vi "Do.vi"(8 "error in (no error)":errorcluster, 10 "Actor in":refnum<class "Actor.lvclass">, 11 "Return Run VI State Msg":refnum<class "Return Run VI State Msg.lvclass">) -> (0 "error out":errorcluster, 2 "Actor out":refnum<class "Actor.lvclass">)   [LabVIEW 2013, in "tWorkerTCPConnection.lvlib" / "Return Run VI State Msg.lvclass"]
doc: "(<B>Filename</B>: Actor Framework.lvlib:Message.lvclass:Do.vi)\n\nDefines what a message does when it is received by an actor. Generally, a message instructs an actor to invoke one of its methods.\n\nBy default, this method does nothing. A child class must override it to define behavior. Create a child class by using the Actor Framework Message Maker dialog box."
uses:
  Return Run VI State Msg.lvclass
  <vilib>/ActorFramework/Actor/Actor.lvclass
  tWorkerTCPConnection/tWorkerTCPConnection.lvclass
  Return Run VI State Msg.lvclass/Return Run VI State Msg.ctl
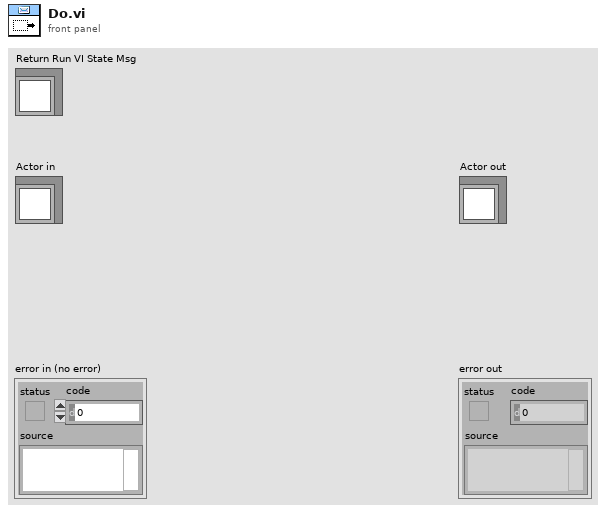
[diagram p1: front panel]
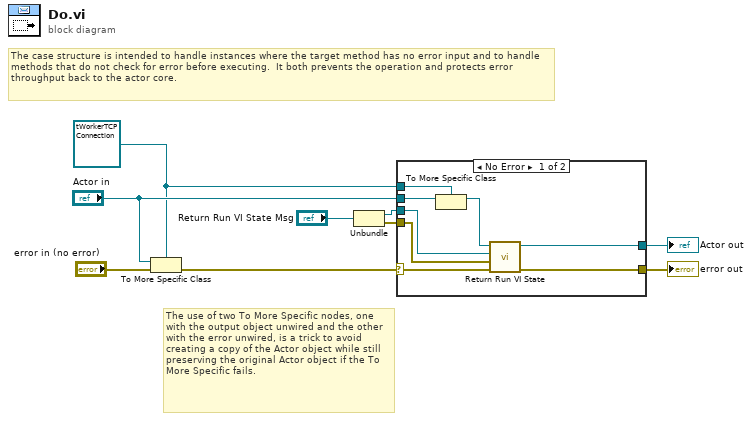
[diagram p0: block diagram]
diagram:
  w1 = refnum<class "tWorkerTCPConnection.lvclass"> refnum ("tWorkerTCPConnection.lvlib:tWorkerTCPConnection.lvclass")
  # "The use of two To More Specific nodes, one with the output object unwired and the other with the error unwired, is a trick to avoid creating a copy of the Actor object while still preserving the original Actor object if the To More Specific fails."
  # "The case structure is intended to handle instances where the target method has no error input and to handle methods that do not check for error before executing.  It both prevents the operation and protects error throughput back to the actor core."
  n1 = To More Specific Class(target class=w1, reference="Actor in", error in="error in (no error)") -> (error out=w9:errorcluster)  [unwired: 1 out]
  n2 = Unbundle("Return Run VI State Msg") -> (w8:refnum<class "tBSONDocument.lvclass">, w7:errorcluster)
  n3 = case shown="No Error" w9 {
    selector: w9 -> [w11 w19]
    tunnel: [w10 w19] -> w2
    tunnel: [w14 w18] -> w3
    tunnel: "Actor in" -> [w16 w18]
    tunnel: w1 -> [w17 _]
    tunnel: w8 -> [w13 _]
    tunnel: w7 -> [w12 _]
    frame No Error {
      n4 = To More Specific Class(target class=w17, reference=w16) -> (specific class reference=w15:refnum<class "tWorkerTCPConnection.lvclass">)  [unwired: 1 in, 1 out]
      n5 = call "Return Run VI State.vi"("error in (no error)"=w11, "Error From Run VI"=w12, "Indicators"=w13, "tWorkerTCPConnection in"=w15) -> ("error out"=w10:errorcluster, "tWorkerTCPConnection out"=w14:refnum<class "tWorkerTCPConnection.lvclass">)  [unwired: 6 in]
    }
    frame Error {
      # "If type check fails, pass the original object out again."
    }
  }
  "error out" <- w2
  "Actor out" <- w3
